vi "Refresh-map-settings.vi"(5 "Active characteristic":T1, 7 "Active camera":T2, 8 "error in":errorcluster, 9 "Read offset buffer in":i64, 10 "Map characteristic buffer in":T1, 11 "Active camer buffer in":T2) -> (0 "error IO":errorcluster, 1 "Read offset":i64, 2 "Map characteristic":T1, 3 "Active camera":T2, 4 "No setting change?":bool)   [LabVIEW 2013, in "CameraVision.lvlib" / "CV-Mapping.lvclass"]
uses:
  CV-Mapping.lvclass
  Mapping-characteristic.ctl
  UI/Camera-selector.ctl
  UI/CV-UI.lvclass
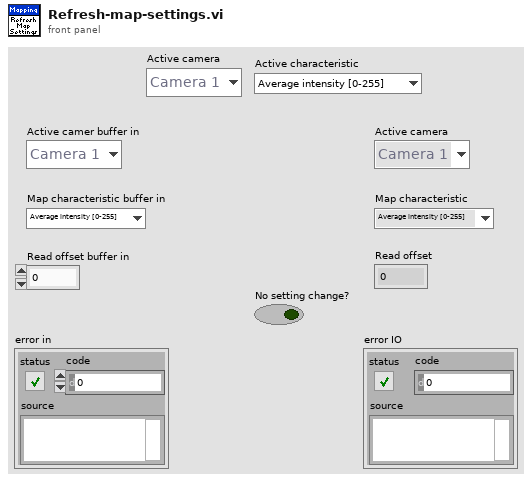
[diagram p1: front panel]
types:
  T1 = typedef "CameraVision.lvlib/CV-Mapping.lvclass/Mapping-characteristic.ctl" = enum16{"Average intensity [0-255]", "Peak intensity [0-255]", "Melt-pool size [mm²]", "Melt-pool aspect ratio []", "Melt-pool fragments []", "Average temperature [°C]", "Max. temperature [°C]", "Min. temperature [°C]", "Std. dev. temperature [°C]"}
  T2 = typedef "CameraVision.lvlib/CV-UI.lvclass/Camera-selector.ctl" = enum16{"Camera 1", "Camera 2"}
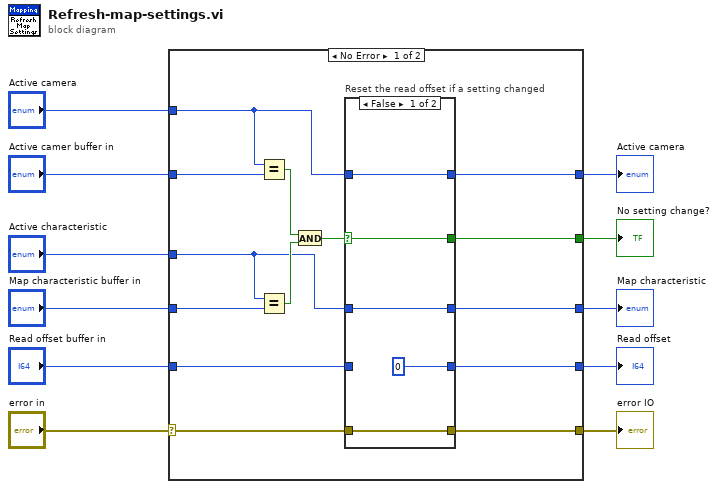
[diagram p0: block diagram]
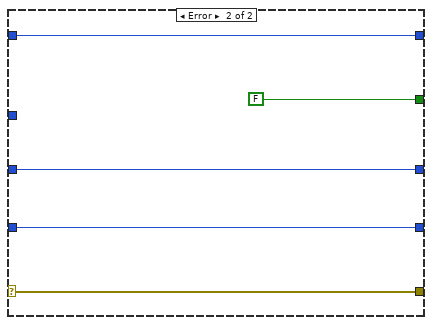
[diagram p3: hidden frame]
diagram:
  n1 = case shown="No Error" "error in" {
    selector: "error in" -> [w12 w40]
    tunnel: [w25 FALSE] -> w11
    tunnel: [w24 w39] -> w10
    tunnel: [w23 w38] -> w9
    tunnel: [w22 w37] -> w8
    tunnel: "Active camer buffer in" -> [w18 w37]
    tunnel: "Read offset buffer in" -> [w17 w39]
    tunnel: "Map characteristic buffer in" -> [w16 w38]
    tunnel: "Active characteristic" -> [w13 _]
    tunnel: [w15 w40] -> w4
    tunnel: "Active camera" -> [w14 _]
    frame No Error {
      n2 = Equal?(x=w14, y=w18) -> (x = y?=w20:bool)
      n3 = Equal?(x=w13, y=w16) -> (x = y?=w21:bool)
      n4 = And(x=w20, y=w21) -> (x .and. y?=w19:bool)
      n5 = case "Reset the read offset if a setting changed" shown="False" w19 {
        selector: w19 -> [w27 w32]
        tunnel: w13 -> [w29 w35]
        tunnel: [w29 w35] -> w23
        tunnel: w17 -> [_ w34]
        tunnel: [i64 0 ("Read offset") w34] -> w24
        tunnel: w14 -> [w28 w33]
        tunnel: [w28 w33] -> w22
        tunnel: [w27 w32] -> w25
        tunnel: w12 -> [w26 w31]
        tunnel: [w26 w31] -> w15
        frame False {
        }
        frame True {
        }
      }
    }
    frame Error {
    }
  }
  "error IO" <- w4
  "No setting change?" <- w11
  "Read offset" <- w10
  "Map characteristic" <- w9
  "Active camera" <- w8
